vi "Write MonochromatorRanges.vi"(8 "error in (no error)":errorcluster, 10 "MonochromatorRanges":T1, 11 "MonoClientCommunicator in":refnum<class "MonoClientCommunicator.lvclass">) -> (0 "error out":errorcluster, 3 "MonoClientCommunicator out":refnum<class "MonoClientCommunicator.lvclass">)   [LabVIEW 2016, in "MonoClientCommunicator.lvclass"]
uses:
  MonoClientCommunicator.lvclass
  Typedefs/MonochromatorRanges.ctl
  MonoClientCommunicator.lvclass/MonoClientCommunicator.ctl
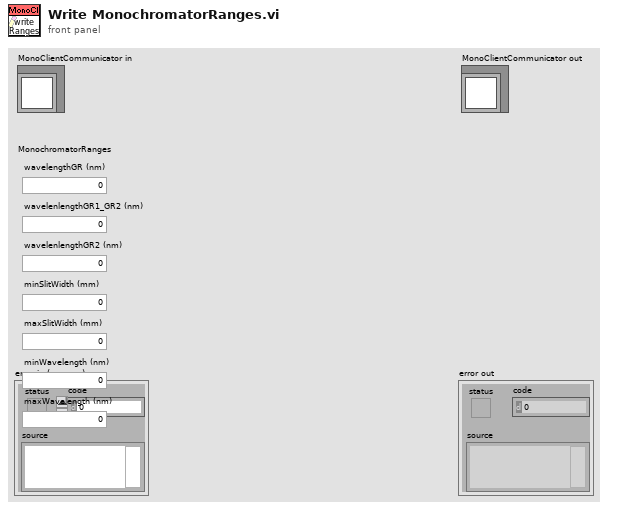
[diagram p1: front panel]
types:
  T1 = typedef "MonochromatorRanges.ctl" = cluster{"maxWavelength (nm)":sgl, "minWavelength (nm)":sgl, "maxSlitWidth (mm)":sgl, "minSlitWidth (mm)":sgl, "wavelenlengthGR2 (nm)":sgl, "wavelenlengthGR1_GR2 (nm)":sgl, "wavelengthGR (nm)":sgl}
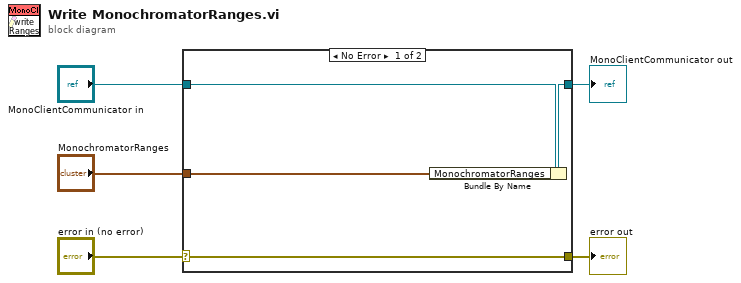
[diagram p0: block diagram]
diagram:
  n1 = case shown="No Error" "error in (no error)" {
    selector: "error in (no error)" -> [w9 w10]
    tunnel: [w9 w10] -> w4
    tunnel: [w7 w11] -> w2
    tunnel: "MonoClientCommunicator in" -> [w8 w11]
    tunnel: "MonochromatorRanges" -> [w6 _]
    frame No Error {
      n2 = Bundle By Name(cluster=w8, "MonochromatorRanges"=w6) -> (w7:refnum<class "MonoClientCommunicator.lvclass">)
    }
    frame Error {
    }
  }
  "error out" <- w4
  "MonoClientCommunicator out" <- w2
